vi "Registro de datos.vi"() -> ()   [LabVIEW 2017]
panel:
  in  "?":bool
  in  "Año de nacimineto":dbl
  out "?":string
  in  "Nombre (s)":string
  in  "Apellido materno":string
  in  "Apellido paterno":string
  # "REGISTRO DE DATOS"
  # "Confirmación de datos"
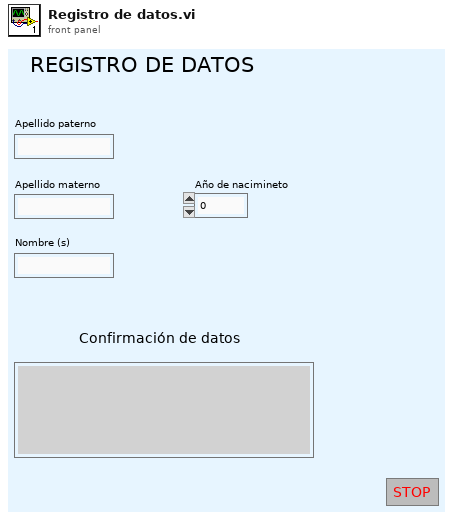
[diagram p1: front panel]
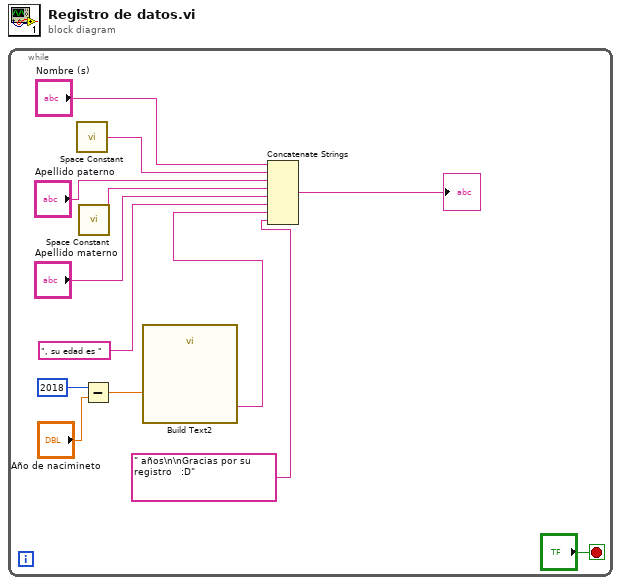
[diagram p0: block diagram]
diagram:
  n1 = while {
    stop <- "?" stop-if-true
    n2 = call <vilib>:"Space Constant.vi"() -> ("String"=w11:string)
    n3 = call <vilib>:"Space Constant.vi"() -> ("String"=w10:string)
    n4 = Subtract(x=2018, y="Año de nacimineto") -> (x-y=w5:dbl)
    n5 = call "Build Text2"("edad"=w5) -> ("Result"=w4:string)  [unwired: 13 in, 1 out]
    n6 = Concatenate Strings("Nombre (s)", w11, "Apellido paterno", w10, "Apellido materno", ", su edad es ", w4, " años\n\nGracias por su registro   :D") -> (→"?":string)
  }
